vi "channel location.vi"(3 "Index":u32, 4 "Sensor Array":T1) -> (1 "Port Location":string)   [LabVIEW 2012]
uses:
  DAQ configuration/Sensor array.ctl
  DAQ configuration/channel identifier.ctl
  DataServer/Server Stats.vi
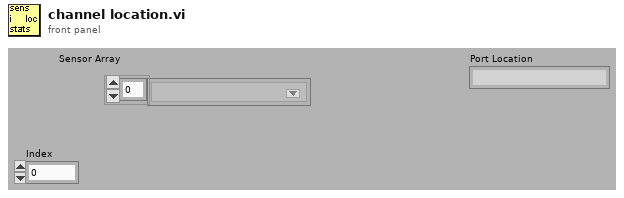
[diagram p1: front panel]
types:
  T1 = typedef "Sensor array.ctl" = T2[]
  T2 = typedef "channel identifier.ctl" = u16
  T3 = typedef "Server stats.ctl" = cluster{"scan rate":dbl, "# connections":i32, "channel settings":cluster{"Name":string, "upper input limits":sgl, "lower input limits":sgl, "Location":string}[]}
  T4 = cluster{"Name":string, "upper input limits":sgl, "lower input limits":sgl, "Location":string}[]
  T5 = cluster{"Name":string, "upper input limits":sgl, "lower input limits":sgl, "Location":string}
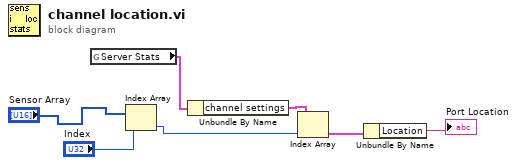
[diagram p0: block diagram]
diagram:
  n1 = global read "Server Stats.vi" "Server Stats"() -> (w6:T3)
  n2 = Index Array(array="Sensor Array", index="Index") -> (element=w3:T2)
  n3 = Unbundle By Name(w6) -> ("channel settings"=w4:T4)
  n4 = Index Array(array=w4, index=w3) -> (element=w2:T5)
  n5 = Unbundle By Name(w2) -> ("Location"=→"Port Location":string)
